vi "Update Status Table by Reference.vi"(8 "error in (no error)":errorcluster, 10 "Plugin Info Array":T1[](array[typedef]) {"Node Status"."Monitor Doubles"."4" format="%#_9g"; "Node Status"."Monitor Doubles"."3" format="%#_9g"; "Node Status"."Monitor Doubles"."2" format="%#_9g"; "Node Status"."Monitor Doubles"."1" format="%#_9g"; "Node Status"."Timing Statistics (us)"."Period"."Avg" format="%_6g"}, 11 "Table Control in":refnum<vi>) -> (0 "error out":errorcluster)   [LabVIEW 2021, in "CIF_UI.lvclass"]
uses:
  CIF_UI.lvclass
  Typedef/PluginInfo.ctl
  Typedef/Version.ctl
  CIFCore/Common/Typedef/gRPC Reported Plugin Status.ctl
  CIFCore/Common/Typedef/Plugin State.ctl
  CIFCore/Common/Typedef/Timing Statistics.ctl
  CIFCore/Common/Typedef/Timing Stats Base.ctl
  CIFCore/Common/Typedef/FIFO Statistics.ctl
  CIFCore/Common/Typedef/Simple Error.ctl
  CIFCore/Common/Typedef/Monitor Doubles.ctl
  CIFCore/Common/Typedef/Monitor U64.ctl
  CIFCore/Common/Typedef/Monitor I64.ctl
  CIF_UI.lvclass/CIF_UI.ctl
  CIFCore/Common/CIFCoreCommon.lvlib
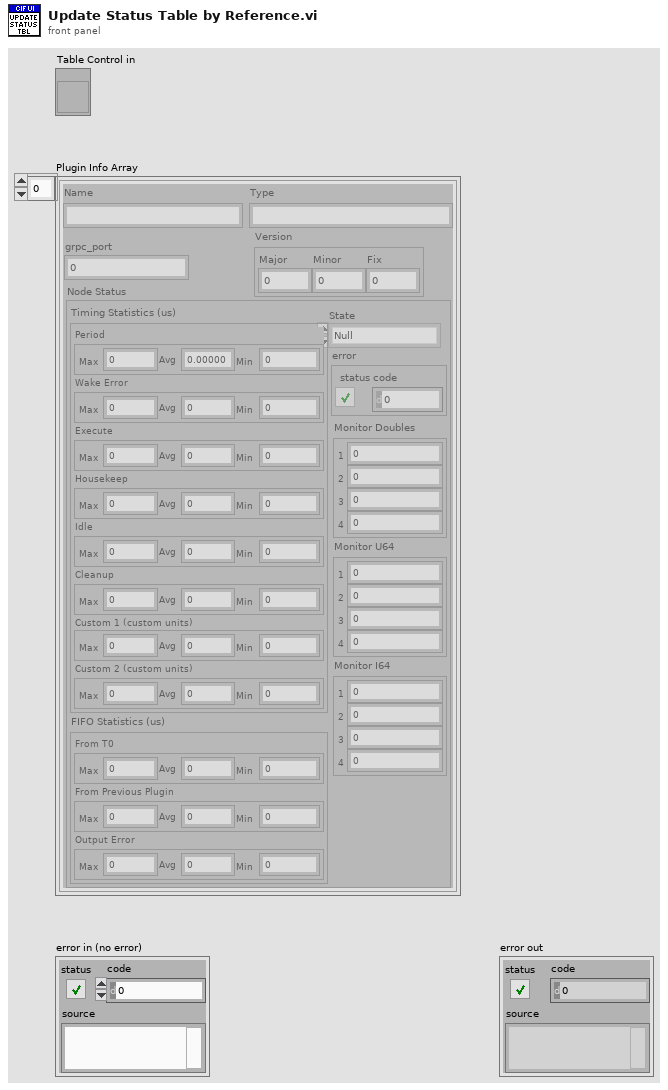
[diagram p1: front panel]
types:
  T1 = typedef "CIF_UI.lvclass/PluginInfo.ctl" = cluster{"Name":string, "Type":string, "grpc_port":i32, "Version":T2, "Node Status":T3}
  T2 = typedef "CIF_UI.lvclass/Version.ctl" = cluster{"Major":i32, "Minor":i32, "Fix":i32}
  T3 = typedef "CIFCoreCommon.lvlib/gRPC Reported Plugin Status.ctl" = cluster{"State":T4, "Timing Statistics (us)":T5, "FIFO Statistics (us)":T7, "error":T8, "Monitor Doubles":T9, "Monitor U64":T10, "Monitor I64":T11}
  T4 = typedef "CIFCoreCommon.lvlib/Plugin State.ctl" = enum32{"Null", "Creating", "Listening", "Running", "CleaningUp", "Destroying"}
  T5 = typedef "CIFCoreCommon.lvlib/Timing Statistics.ctl" = cluster{"Period":T6, "Wake Error":T6, "Execute":T6, "Housekeep":T6, "Idle":T6, "Cleanup":T6, "Custom 1 (custom units)":T6, "Custom 2 (custom units)":T6}
  T6 = typedef "CIFCoreCommon.lvlib/Timing Stats Base.ctl" = cluster{"Max":i64, "Avg":dbl, "Min":i64}
  T7 = typedef "CIFCoreCommon.lvlib/FIFO Statistics.ctl" = cluster{"From T0":T6, "From Previous Plugin":T6, "Output Error":T6}
  T8 = typedef "CIFCoreCommon.lvlib/Simple Error.ctl" = cluster{"status":bool, "code":i32}
  T9 = typedef "CIFCoreCommon.lvlib/Monitor Doubles.ctl" = cluster{"1":dbl, "2":dbl, "3":dbl, "4":dbl}
  T10 = typedef "CIFCoreCommon.lvlib/Monitor U64.ctl" = cluster{"1":u64, "2":u64, "3":u64, "4":u64}
  T11 = typedef "CIFCoreCommon.lvlib/Monitor I64.ctl" = cluster{"1":i64, "2":i64, "3":i64, "4":i64}
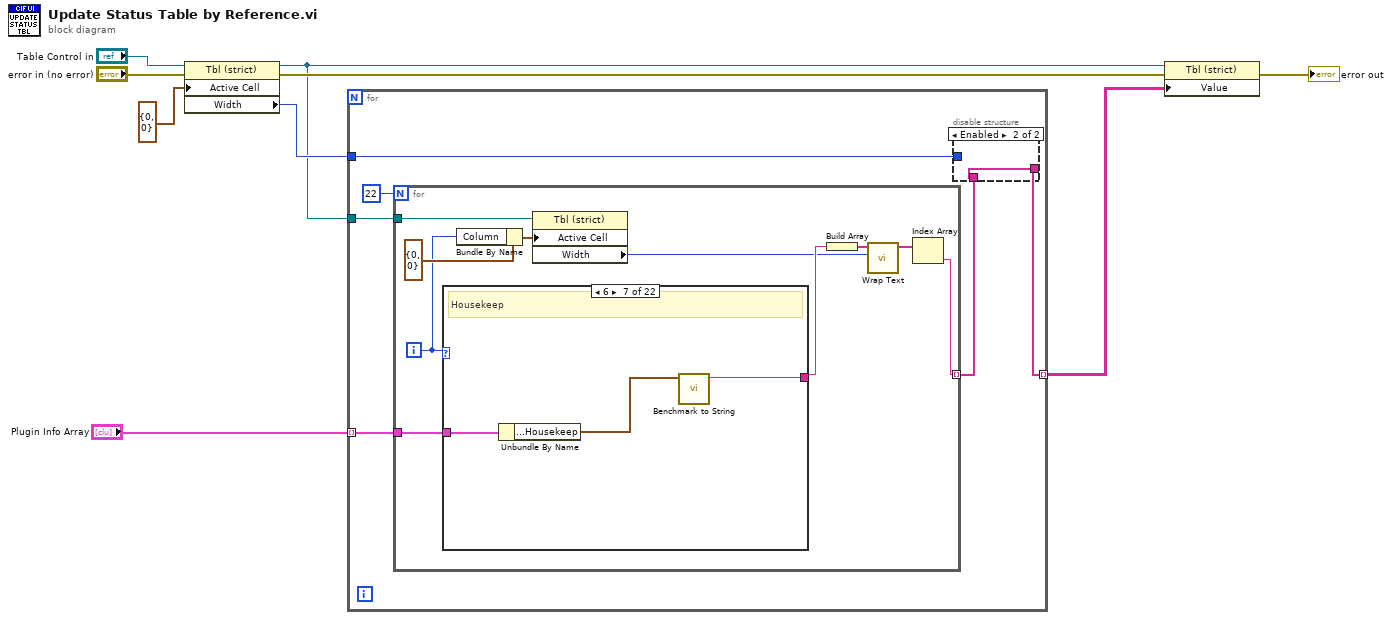
[diagram p0: block diagram]
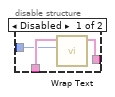
[diagram p2: hidden frame]
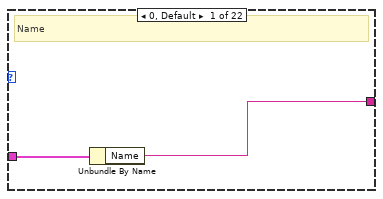
[diagram p3: hidden frame]
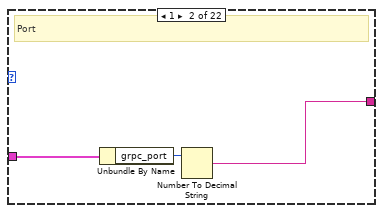
[diagram p4: hidden frame]
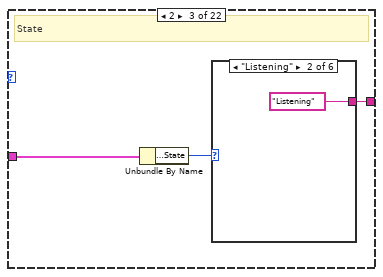
[diagram p5: hidden frame]
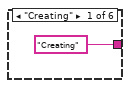
[diagram p6: hidden frame]
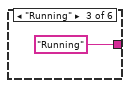
[diagram p7: hidden frame]
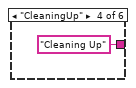
[diagram p8: hidden frame]
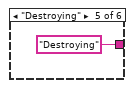
[diagram p9: hidden frame]
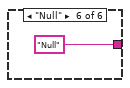
[diagram p10: hidden frame]
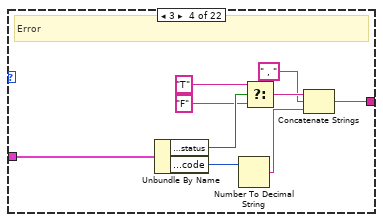
[diagram p11: hidden frame]
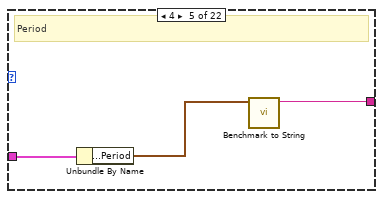
[diagram p12: hidden frame]
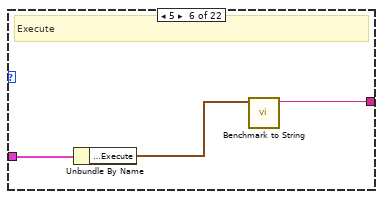
[diagram p13: hidden frame]
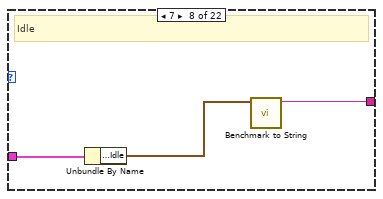
[diagram p14: hidden frame]
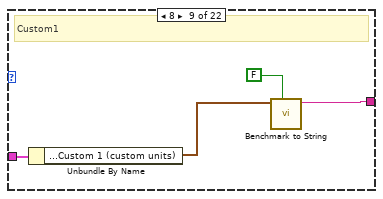
[diagram p15: hidden frame]
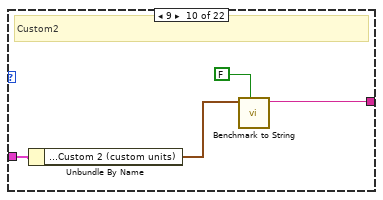
[diagram p16: hidden frame]
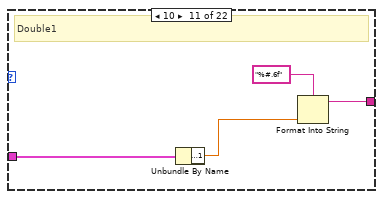
[diagram p17: hidden frame]
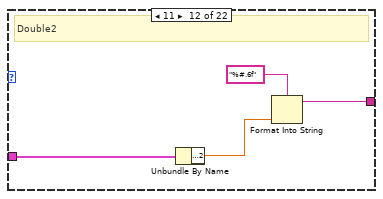
[diagram p18: hidden frame]
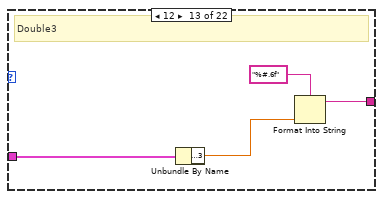
[diagram p19: hidden frame]
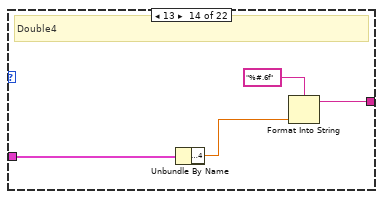
[diagram p20: hidden frame]
diagram:
  n1 = property on="Property Node" class="Tbl (strict)"(reference="Table Control in", error in="error in (no error)", "Active Cell"=cluster{"Row":i32, "Column":i32} {"Row"=0, "Column"=0}) -> (reference out=w2:refnum<vi>, error out=w6:errorcluster, "Width"=w4:u32)
  n2 = for {
    tunnel: [w12] -> w3 mode=indexing
    tunnel: "Plugin Info Array" -> [w14] mode=indexing
    tunnel: w4 -> [w11]
    tunnel: w2 -> [w10]
    n3 = for {
      N: 22 -> [_]
      tunnel: [w25] -> w13 mode=indexing
      tunnel: w14 -> [w29]
      tunnel: w10 -> [w24]
      i -> [w22]
      n4 = case shown="6" w22 {
        tunnel: [w30 w34 w35 w44 w54 w57 w60 w63 w67 w70 w73 w78 w82 w86 w89 w92 w95 w98 w101 w104 w107 w110] -> w26
        tunnel: w29 -> [w31 w33 w37 w52 w55 w58 w61 w64 w68 w72 w76 w80 w84 w88 w91 w94 w97 w100 w103 w106 w109 w112]
        frame 0, Default {
          # "Name"
          n5 = Unbundle By Name(w31) -> ("Name"=w30:string)
        }
        frame 1 {
          # "Port"
          n6 = Unbundle By Name(w33) -> ("grpc_port"=w32:i32)
          n7 = Number To Decimal String(number=w32) -> (decimal integer string=w34:string)  [unwired: 1 in]
        }
        frame 2 {
          # "State"
          n8 = Unbundle By Name(w37) -> ("Node Status.State"=w36:T4)
          n9 = case shown="\"Listening\"" w36 {
            tunnel: ["Creating" "Listening" "Running" "Cleaning Up" "Destroying" "Null"] -> w35
            frame "Creating" {
            }
            frame "Listening" {
            }
            frame "Running" {
            }
            frame "CleaningUp" {
            }
            frame "Destroying" {
            }
            frame "Null" {
            }
          }
        }
        frame 3 {
          # "Error"
          n10 = Unbundle By Name(w52) -> ("Node Status.error.status"=w50:bool, "Node Status.error.code"=w51:i32)
          n11 = Number To Decimal String(number=w51) -> (decimal integer string=w45:string)  [unwired: 1 in]
          n12 = Select(t="T", s=w50, f="F") -> (s? t:f=w47:string)
          n13 = Concatenate Strings(w47, " , ", w45) -> (w44:string)
        }
        frame 4 {
          # "Period"
          n14 = Unbundle By Name(w55) -> ("Node Status.Timing Statistics (us).Period"=w53:T6)
          n15 = call "Benchmark to String.vi"("Timing Stats"=w53) -> ("concatenated string"=w54:string)  [unwired: 10 in]
        }
        frame 5 {
          # "Execute"
          n16 = Unbundle By Name(w58) -> ("Node Status.Timing Statistics (us).Execute"=w56:T6)
          n17 = call "Benchmark to String.vi"("Timing Stats"=w56) -> ("concatenated string"=w57:string)  [unwired: 10 in]
        }
        frame 6 {
          # "Housekeep"
          n18 = Unbundle By Name(w61) -> ("Node Status.Timing Statistics (us).Housekeep"=w59:T6)
          n19 = call "Benchmark to String.vi"("Timing Stats"=w59) -> ("concatenated string"=w60:string)  [unwired: 10 in]
        }
        frame 7 {
          # "Idle"
          n20 = Unbundle By Name(w64) -> ("Node Status.Timing Statistics (us).Idle"=w62:T6)
          n21 = call "Benchmark to String.vi"("Timing Stats"=w62) -> ("concatenated string"=w63:string)  [unwired: 10 in]
        }
        frame 8 {
          # "Custom1"
          n22 = Unbundle By Name(w68) -> ("Node Status.Timing Statistics (us).Custom 1 (custom units)"=w66:T6)
          n23 = call "Benchmark to String.vi"("Divide/1k"=FALSE, "Timing Stats"=w66) -> ("concatenated string"=w67:string)  [unwired: 9 in]
        }
        frame 9 {
          # "Custom2"
          n24 = Unbundle By Name(w72) -> ("Node Status.Timing Statistics (us).Custom 2 (custom units)"=w71:T6)
          n25 = call "Benchmark to String.vi"("Divide/1k"=FALSE, "Timing Stats"=w71) -> ("concatenated string"=w70:string)  [unwired: 9 in]
        }
        frame 10 {
          # "Double1"
          n26 = Unbundle By Name(w76) -> ("Node Status.Monitor Doubles.1"=w74:dbl)
          n27 = Format Into String(format string="%#.6f", w74) -> (resulting string=w73:string)  [unwired: 2 in, 1 out]
        }
        frame 11 {
          # "Double2"
          n28 = Unbundle By Name(w80) -> ("Node Status.Monitor Doubles.2"=w77:dbl)
          n29 = Format Into String(format string="%#.6f", w77) -> (resulting string=w78:string)  [unwired: 2 in, 1 out]
        }
        frame 12 {
          # "Double3"
          n30 = Unbundle By Name(w84) -> ("Node Status.Monitor Doubles.3"=w81:dbl)
          n31 = Format Into String(format string="%#.6f", w81) -> (resulting string=w82:string)  [unwired: 2 in, 1 out]
        }
        frame 13 {
          # "Double4"
          n32 = Unbundle By Name(w88) -> ("Node Status.Monitor Doubles.4"=w85:dbl)
          n33 = Format Into String(format string="%#.6f", w85) -> (resulting string=w86:string)  [unwired: 2 in, 1 out]
        }
        frame 14 {
          # "U64_1"
          n34 = Unbundle By Name(w91) -> ("Node Status.Monitor U64.1"=w90:u64)
          n35 = Number To Decimal String(number=w90) -> (decimal integer string=w89:string)  [unwired: 1 in]
        }
        frame 15 {
          # "U64_2"
          n36 = Unbundle By Name(w94) -> ("Node Status.Monitor U64.2"=w93:u64)
          n37 = Number To Decimal String(number=w93) -> (decimal integer string=w92:string)  [unwired: 1 in]
        }
        frame 16 {
          # "U64_3"
          n38 = Unbundle By Name(w97) -> ("Node Status.Monitor U64.3"=w96:u64)
          n39 = Number To Decimal String(number=w96) -> (decimal integer string=w95:string)  [unwired: 1 in]
        }
        frame 17 {
          # "U64_4"
          n40 = Unbundle By Name(w100) -> ("Node Status.Monitor U64.4"=w99:u64)
          n41 = Number To Decimal String(number=w99) -> (decimal integer string=w98:string)  [unwired: 1 in]
        }
        frame 18 {
          # "I64_1"
          n42 = Unbundle By Name(w103) -> ("Node Status.Monitor I64.1"=w102:i64)
          n43 = Number To Decimal String(number=w102) -> (decimal integer string=w101:string)  [unwired: 1 in]
        }
        frame 19 {
          # "I64_2"
          n44 = Unbundle By Name(w106) -> ("Node Status.Monitor I64.2"=w105:i64)
          n45 = Number To Decimal String(number=w105) -> (decimal integer string=w104:string)  [unwired: 1 in]
        }
        frame 20 {
          # "I64_3"
          n46 = Unbundle By Name(w109) -> ("Node Status.Monitor I64.3"=w108:i64)
          n47 = Number To Decimal String(number=w108) -> (decimal integer string=w107:string)  [unwired: 1 in]
        }
        frame 21 {
          # "I64_4"
          n48 = Unbundle By Name(w112) -> ("Node Status.Monitor I64.4"=w111:i64)
          n49 = Number To Decimal String(number=w111) -> (decimal integer string=w110:string)  [unwired: 1 in]
        }
      }
      n50 = Bundle By Name(cluster=cluster{"Row":i32, "Column":i32} {"Row"=0, "Column"=0} ("Active Cell"), "Column"=w22) -> (w20:cluster{"Row":i32, "Column":i32})
      n51 = property on="Property Node" class="Tbl (strict)"(reference=w24, "Active Cell"=w20) -> ("Width"=w21:u32)  [unwired: 1 in, 2 out]
      n52 = Build Array(w26) -> (w28:string[])
      n53 = call "Wrap Text.vi"("width"=w21, "item names"=w28) -> ("item names with wrapping"=w27:string[])  [unwired: 8 in, 1 out]
      n54 = Index Array(array=w27) -> (element=w25:string)  [unwired: 1 in]
    }
    n55 = disable-structure shown="Enabled" {
      disable-tunnel: w13 -> [w18 w19]
      disable-tunnel: [w17 w19] -> w12
      disable-tunnel: w11 -> [w16 _]
      frame Disabled {
        n56 = call "Wrap Text.vi"("width"=w16, "item names"=w18) -> ("item names with wrapping"=w17:string[])  [unwired: 8 in, 1 out]
      }
      frame Enabled {
      }
    }
  }
  n57 = property class="Tbl (strict)"(reference=w2, error in=w6, "Value"=w3) -> (error out=→"error out":errorcluster)  [unwired: 1 out]
